vi "sub_apt_movejog.vi"(8 "错误输入（无错误）":errorcluster, 9 "Rel. Pos Y":dbl=0.05 min=-10.0 max=360.0 format="%.4f", 10 "lJogDir":i32, 11 "引用":refnum<k7>) -> (0 "error out":errorcluster, 3 "MG17Motor Y":refnum<k7>)   [LabVIEW 2015]
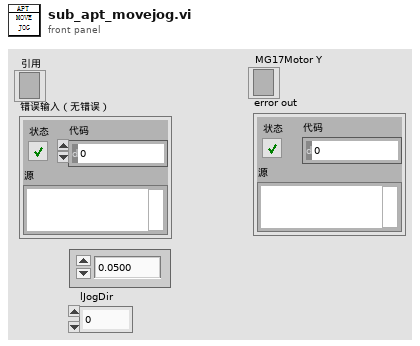
[diagram p1: front panel]
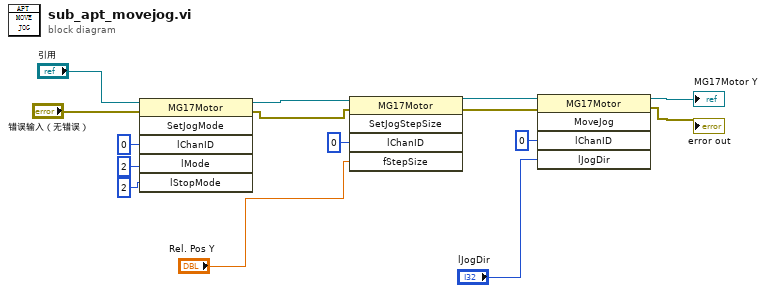
[diagram p0: block diagram]
diagram:
  n1 = invoke class="MG17Motor" method="SetJogMode"(reference="引用", error in="错误输入（无错误）", "lChanID"=0, "lMode"=2, "lStopMode"=2) -> (reference out=w11:refnum<k7>, error out=w12:errorcluster)  [unwired: 1 in, 4 out]
  n2 = invoke class="MG17Motor" method="SetJogStepSize"(reference=w11, error in=w12, "lChanID"=0, "fStepSize"="Rel. Pos Y") -> (reference out=w5:refnum<k7>, error out=w2:errorcluster)  [unwired: 1 in, 3 out]
  n3 = invoke class="MG17Motor" method="MoveJog"(reference=w5, error in=w2, "lChanID"=0, "lJogDir"="lJogDir") -> (reference out=→"MG17Motor Y":refnum<k7>, error out=→"error out":errorcluster)  [unwired: 1 in, 3 out]
